vi "Test Shield Communication.vi"(8 "error in (no error)":errorcluster, 11 "Arduino Shield in":refnum<class "Arduino Shield.lvclass">) -> (0 "error out":errorcluster, 3 "Arduino Shield out":refnum<class "Arduino Shield.lvclass">)   [LabVIEW 2020, in "Arduino Shield.lvclass"]
uses:
  Arduino Shield.lvclass
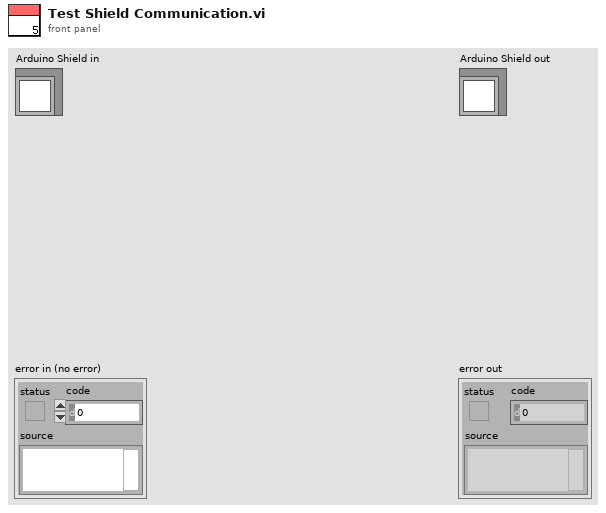
[diagram p1: front panel]
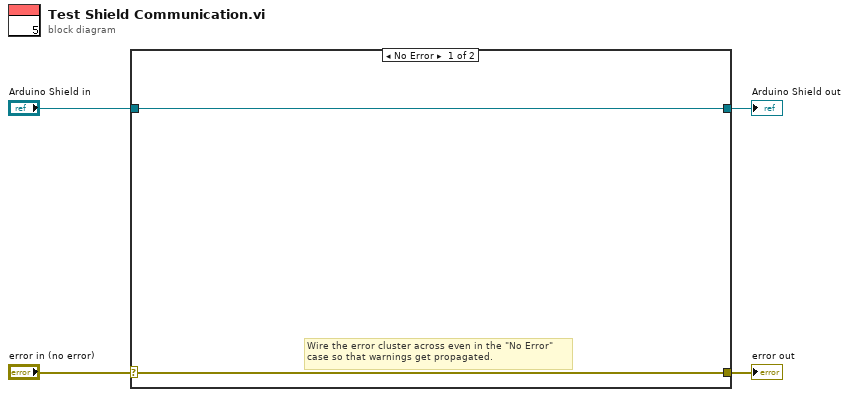
[diagram p0: block diagram]
diagram:
  n1 = case shown="No Error" "error in (no error)" {
    selector: "error in (no error)" -> [w5 w8]
    tunnel: [w5 w8] -> w3
    tunnel: [w6 w7] -> w1
    tunnel: "Arduino Shield in" -> [w6 w7]
    frame No Error {
      # "Wire the error cluster across even in the \"No Error\"\ncase so that warnings get propagated."
    }
    frame Error {
    }
  }
  "error out" <- w3
  "Arduino Shield out" <- w1
